vi "WriteBodeRow.vi"(7 "Frequency (Hz)":i32, 8 "error in (no error)":errorcluster, 9 "Gain (dB)":dbl, 10 "Wrapped\nPhase\nDifference\n(-180,180]":dbl, 11 "File RefNum in":refnum<file>) -> (0 "error out":errorcluster, 3 "File RefNum out":refnum<file>)   [LabVIEW 2026]
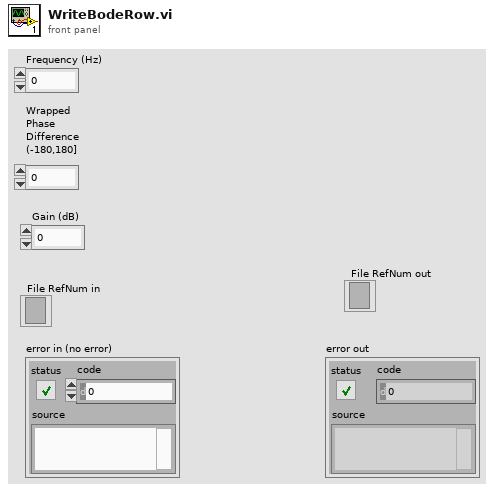
[diagram p1: front panel]
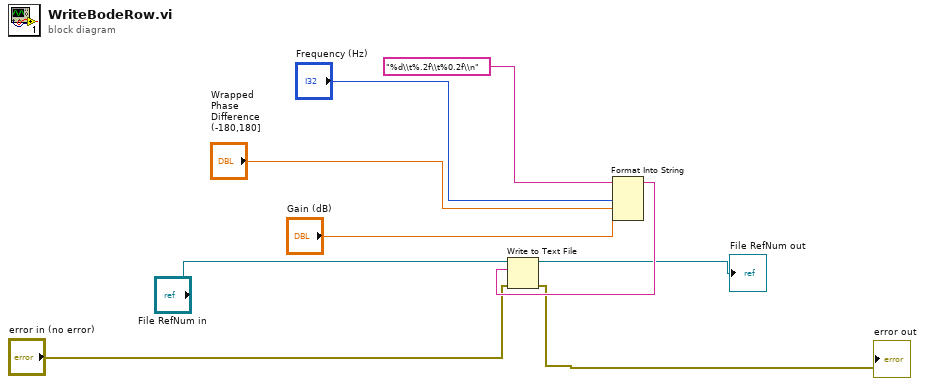
[diagram p0: block diagram]
diagram:
  n1 = Format Into String(format string="%d\\t%.2f\\t%0.2f\\n", "Frequency (Hz)", "Wrapped\nPhase\nDifference\n(-180,180]", "Gain (dB)") -> (resulting string=w9:string)  [unwired: 2 in, 1 out]
  n2 = Write to Text File(file (use dialog)="File RefNum in", text=w9, error in="error in (no error)") -> (refnum out=→"File RefNum out":refnum<file>, error out=→"error out":errorcluster)  [unwired: 1 in, 1 out]
